vi "send_data.vi"(8 "error in (no error)":errorcluster, 10 "data variant":variant, 11 "StreamingBase in":refnum<class "StreamingBase.lvclass">) -> (0 "error out":errorcluster, 3 "StreamingBase out":refnum<class "StreamingBase.lvclass">)   [LabVIEW 2011, in "StreamingBase.lvclass"]
uses:
  StreamingBase.lvclass
  StreamingBase.lvclass/StreamingBase.ctl
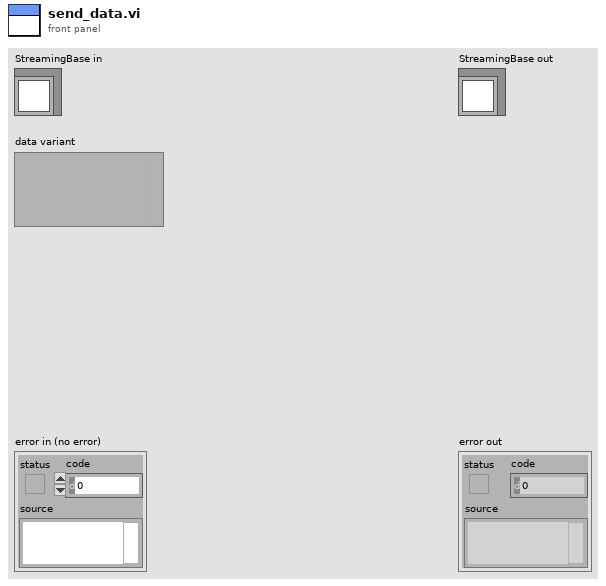
[diagram p1: front panel]
types:
  T1 = typedef "StreamingBase.lvclass/observer_cluster.ctl" = cluster{"writer endpoint":refnum<k21>, "reader endpoint":refnum<k21>}
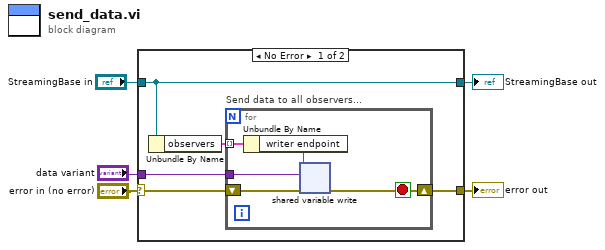
[diagram p0: block diagram]
diagram:
  n1 = case shown="No Error" "error in (no error)" {
    selector: "error in (no error)" -> [w9 w17]
    tunnel: [w8 w17] -> w4
    tunnel: [w10 w16] -> w2
    tunnel: "StreamingBase in" -> [w10 w16]
    tunnel: "data variant" -> [w6 _]
    frame No Error {
      n2 = Unbundle By Name(w10) -> ("observers"=w7:T1[])
      n3 = for "Send data to all observers..." {
        shift-right: [w12] -> w8
        shift-left: w9 -> [w13]
        tunnel: w7 -> [w15] mode=indexing
        tunnel: w6 -> [w11]
        stop <- w12 stop-if-true
        n4 = Unbundle By Name(w15) -> ("writer endpoint"=w14:refnum<k21>)
        n5 = shared-variable-write(w14, w13, w11) -> (w12:errorcluster)  [unwired: 1 in, 2 out]
      }
    }
    frame Error {
    }
  }
  "error out" <- w4
  "StreamingBase out" <- w2
